vi "FTDI_MPSSE_Ini.vi"(10 "Channel Nmb":u8) -> (0 "error out":errorcluster, 1 "Serial number":string, 2 "Ini Status":bool, 3 "Handler":u32, 5 "Description":string)   [LabVIEW 2018]
uses:
  dll/libMPSSE.dll
  libMPSSE-SPI.lvlib
panel:
  out "Flags":u32 format="%b"
  out "Type":u32
  out "ID":u32 format="%08x"
  out "LocId":u32
  out "ftHandle":u32 format="%08x"
  out "numChannels":i32
  # "FTDI Info"
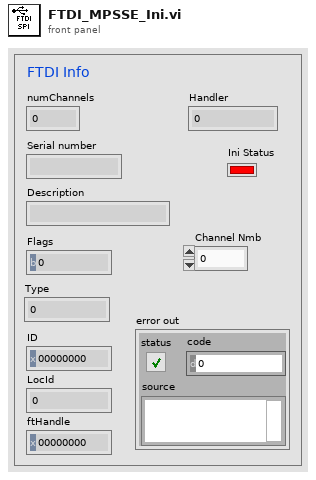
[diagram p1: front panel]
types:
  T1 = cluster{"Flags":u32, "Type":u32, "ID":u32, "LocId":u32, "SerialNumber[0]":i8, "SerialNumber[1]":i8, "SerialNumber[2]":i8, "SerialNumber[3]":i8, "SerialNumber[4]":i8, "SerialNumber[5]":i8, "SerialNumber[6]":i8, "SerialNumber[7]":i8, "SerialNumber[8]":i8, "SerialNumber[9]":i8, "SerialNumber[10]":i8, "SerialNumber[11]":i8, "SerialNumber[12]":i8, "SerialNumber[13]":i8, "SerialNumber[14]":i8, "SerialNumber[15]":i8, "Description[0]":i8, "Description[1]":i8, "Description[2]":i8, "Description[3]":i8, "Description[4]":i8, "Description[5]":i8, "Description[6]":i8, "Description[7]":i8, "Description[8]":i8, "Description[9]":i8, "Description[10]":i8, "Description[11]":i8, "Description[12]":i8, "Description[13]":i8, "Description[14]":i8, "Description[15]":i8, "Description[16]":i8, "Description[17]":i8, "Description[18]":i8, "Description[19]":i8, "Description[20]":i8, "Description[21]":i8, "Description[22]":i8, "Description[23]":i8, "Description[24]":i8, "Description[25]":i8, "Description[26]":i8, "Description[27]":i8, "Description[28]":i8, "Description[29]":i8, "Description[30]":i8, "Description[31]":i8, "Description[32]":i8, "Description[33]":i8, "Description[34]":i8, "Description[35]":i8, "Description[36]":i8, "Description[37]":i8, "Description[38]":i8, "Description[39]":i8, "Description[40]":i8, "Description[41]":i8, "Description[42]":i8, "Description[43]":i8, "Description[44]":i8, "Description[45]":i8, "Description[46]":i8, "Description[47]":i8, "Description[48]":i8, "Description[49]":i8, "Description[50]":i8, "Description[51]":i8, "Description[52]":i8, "Description[53]":i8, "Description[54]":i8, "Description[55]":i8, "Description[56]":i8, "Description[57]":i8, "Description[58]":i8, "Description[59]":i8, "Description[60]":i8, "Description[61]":i8, "Description[62]":i8, "Description[63]":i8, "ftHandle":u32}
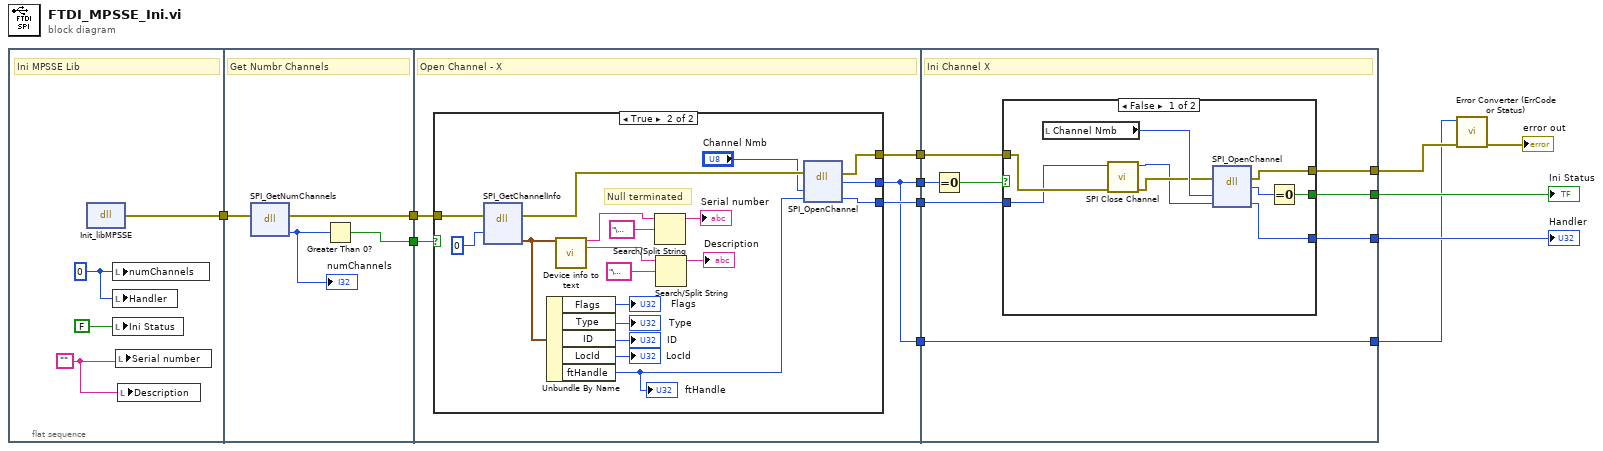
[diagram p0: block diagram]
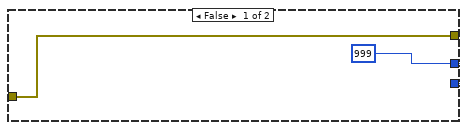
[diagram p2: hidden frame]
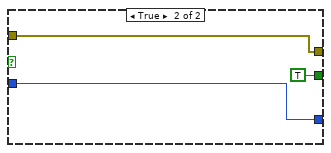
[diagram p3: hidden frame]
diagram:
  n1 = flat-sequence {
    tunnel: [w16] -> w12
    tunnel: w12 -> [w20]
    tunnel: [w19] -> w11
    tunnel: [w17] -> w10
    tunnel: w11 -> [w25]
    tunnel: w10 -> [w24]
    tunnel: [w21] -> w9
    tunnel: [w23] -> w8
    tunnel: [w22] -> w7
    tunnel: [w21] -> w1
    tunnel: w9 -> [w54]
    tunnel: w8 -> [w53]
    tunnel: w7 -> [w52]
    tunnel: [w51] -> w5
    tunnel: [w50] -> w6
    tunnel: [w49] -> w3
    tunnel: [w48] -> w2
    tunnel: w1 -> [w48]
    frame #0 {
      w13 = ""
      w15 = 0 ("numChannels")
      # "Ini MPSSE Lib"
      n2 = dll-call lib="D:/LABVIEW/Examples - 32bit/FTDI/libMPSSE-SPI-LabVIEW-master SNA v3/dll/libMPSSE.dll" fn="Init_libMPSSE"() -> (error out=w16:errorcluster)  [unwired: 4 in, 1 out]
      n3 = local write "numChannels"(w15) -> ()
      n4 = local write "Handler"(w15) -> ()
      n5 = local write "Ini Status"(FALSE ("Ini Status")) -> ()
      n6 = local write "Serial number"(w13) -> ()
      n7 = local write "Description"(w13) -> ()
    }
    frame #1 {
      # "Get Numbr Channels"
      n8 = dll-call lib="D:/LABVIEW/Examples - 32bit/FTDI/libMPSSE-SPI-LabVIEW-master SNA v3/dll/libMPSSE.dll" fn="SPI_GetNumChannels"(error in=w20) -> (error out=w19:errorcluster, "numChannels"=w18:i32)  [unwired: 4 in, 1 out]
      "numChannels" <- w18
      n9 = Greater Than 0?(x=w18) -> (x > 0?=w17:bool)
    }
    frame #2 {
      # "Open Channel - X"
      n10 = case shown="True" w24 {
        tunnel: w25 -> [w26 w41]
        tunnel: [w27 w38] -> w21
        tunnel: [w27 w37] -> w22
        tunnel: [w26 w36] -> w23
        frame False {
          w27 = u32 999 ("return type")
        }
        frame True {
          # "Null terminated"
          n11 = dll-call lib="D:/LABVIEW/Examples - 32bit/FTDI/libMPSSE-SPI-LabVIEW-master SNA v3/dll/libMPSSE.dll" fn="SPI_GetChannelInfo"(error in=w41, "index"=0) -> (error out=w39:errorcluster, "chanInfo out"=w46:T1)  [unwired: 5 in, 1 out]
          n12 = Unbundle By Name(w46) -> ("Flags"=→"Flags":u32, "Type"=→"Type":u32, "ID"=→"ID":u32, "LocId"=→"LocId":u32, "ftHandle"=w29:u32)
          "ftHandle" <- w29
          n13 = call "Device info to text.vi"("chanInfo out"=w46) -> ("Serial number"=w43:string, "Description"=w42:string)  [unwired: 13 in]
          n14 = Search/Split String(string=w43, search string/char (-)="\u0000") -> (substring before match=→"Serial number":string)  [unwired: 1 in, 2 out]
          n15 = Search/Split String(string=w42, search string/char (-)="\u0000") -> (substring before match=→"Description":string)  [unwired: 1 in, 2 out]
          n16 = dll-call lib="D:/LABVIEW/Examples - 32bit/FTDI/libMPSSE-SPI-LabVIEW-master SNA v3/dll/libMPSSE.dll" fn="SPI_OpenChannel"(error in=w39, "index"="Channel Nmb", "handle"=w29) -> (error out=w36:errorcluster, "return type"=w38:u32, "handle"=w37:u32)  [unwired: 3 in, 1 out]
        }
      }
    }
    frame #3 {
      # "Ini Channel X"
      n17 = Equal To 0?(x=w54) -> (x = 0?=w47:bool)
      n18 = case shown="False" w47 {
        tunnel: w52 -> [w56 w65]
        tunnel: w53 -> [w58 w64]
        tunnel: [w63 TRUE] -> w50
        tunnel: [w59 w65] -> w51
        tunnel: [w61 w64] -> w49
        frame False {
          n19 = local read "Channel Nmb"() -> (w60:u8)
          n20 = call "SPI Close Channel.vi"("error in (no error)"=w58, "handle"=w56) -> ("error out"=w57:errorcluster, "handle out"=w55:u32)  [unwired: 7 in, 1 out]
          n21 = dll-call lib="D:/LABVIEW/Examples - 32bit/FTDI/libMPSSE-SPI-LabVIEW-master SNA v3/dll/libMPSSE.dll" fn="SPI_OpenChannel"(error in=w57, "index"=w60, "handle"=w55) -> (error out=w61:errorcluster, "return type"=w62:u32, "handle"=w59:u32)  [unwired: 3 in, 1 out]
          n22 = Equal To 0?(x=w62) -> (x = 0?=w63:bool)
        }
        frame True {
        }
      }
    }
  }
  n23 = call "Error Converter (ErrCode or Status).vi"("error in (no error)"=w3, "error code"=w2) -> ("error out"=→"error out":errorcluster)  [unwired: 9 in]
  "Handler" <- w5
  "Ini Status" <- w6
